vi "Update HDF5 Tree Group Icons.vi"(8 "error in":errorcluster, 10 "Tree":refnum<vi>) -> (0 "error out":errorcluster, 2 "Tree out":refnum<vi>)   [LabVIEW 2017]
doc: "Populates a LabVIEW tree control with the contents of an HDF5 file."
uses:
  <vilib>/UPVI/lvhdf5/utility.llb/private/TreeIconsEnum.ctl
panel:
  # "LVHDF5 Toolkit\nCopyright (c) 2005-2013 by Jason D. Sommerville\nCopyright (c) 2014 by UPVI, LLC.\n\nThis use and distribution of this file is governed by the terms found in \nLICENSE.txt distributed with this toolkit and installed at\n <user.lib>\\_lvhdf5\\LICENSE.txt"
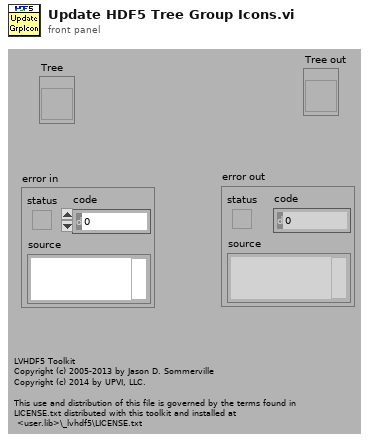
[diagram p1: front panel]
types:
  T1 = typedef "TreeIconsEnum.ctl" = enum16{"None", "Closed Group", "Open Group", "Array Dataset", "Compound Dataset", "Datatype"}
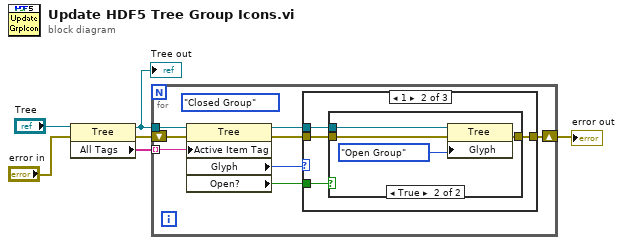
[diagram p0: block diagram]
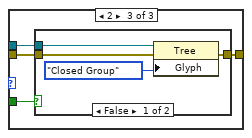
[diagram p4: hidden frame]
diagram:
  n1 = property class="Tree"(reference="Tree", error in="error in") -> (reference out=w3:refnum<vi>, error out=w2:errorcluster, "All Tags"=w4:string[])
  "Tree out" <- w3
  n2 = for {
    tunnel: w4 -> [w13] mode=indexing
    tunnel: w3 -> [w14]
    shift-right: [w7] -> w1
    shift-left: w2 -> [w8]
    (unwired) TreeIconsEnum."Closed Group" ("TreeIcons")
    n3 = property class="Tree"(reference=w14, error in=w8, "Active Item Tag"=w13) -> (reference out=w12:refnum<vi>, error out=w11:errorcluster, "Glyph"=w10:i32, "Open?"=w9:bool)
    n4 = case shown="1" w10 {
      tunnel: w12 -> [_ w19 w28]
      tunnel: w11 -> [w15 w18 w27]
      tunnel: w9 -> [_ w17 w26]
      tunnel: [w15 w16 w25] -> w7
      frame 0, Default {
      }
      frame 1 {
        n5 = case shown="True" w17 {
          tunnel: w19 -> [_ w24]
          tunnel: w18 -> [w20 w23]
          tunnel: [w20 w21] -> w16
          frame False {
          }
          frame True {
            n6 = property class="Tree"(reference=w24, error in=w23, "Glyph"=TreeIconsEnum."Open Group" ("TreeIcons")) -> (error out=w21:errorcluster)  [unwired: 1 out]
          }
        }
      }
      frame 2 {
        n7 = case shown="False" w26 {
          tunnel: w28 -> [w32 _]
          tunnel: w27 -> [w31 w33]
          tunnel: [w29 w33] -> w25
          frame False {
            n8 = property class="Tree"(reference=w32, error in=w31, "Glyph"=TreeIconsEnum."Closed Group" ("TreeIcons")) -> (error out=w29:errorcluster)  [unwired: 1 out]
          }
          frame True {
          }
        }
      }
    }
  }
  "error out" <- w1
